vi "setup-cs-scan-fpga.vi"(4 "state-machine-params":T5={"xy_settled_samples_threshold"=15, "xy_error_threshold"=0.01, "zup_err_threshold"=0.10000228881835938, "prescan_samples"=5000, "TOL"=0.3, "collect_all"=TRUE, "numEntities"=0} {"TOL" format="%#_13g"}, 5 "Control-matrices":sgl[](array[numeric]), 6 "log-channels":u16(ring) items=["without-friction"=5, "with-friction"=6], 7 "ControlParamsLin-ss":T2={"umax"=3.0, "Ns_obs/cntrl"=0, "du_max"=0.0, "Nbar"=0.0, "Nhyst"=0, "Nsat"=0, "Ndrift+1"=0, "Ki-y"=0.01, "Ns_xff+1"=0, "Ns_yff+1"=0, "Ns_Dx+1"=0, "Ns_Dy+1"=0, "Ki-x"=0.01}, 8 "error in":errorcluster, 10 "z_axis_params":T3={"z_u_max"=5.0, "setpoint_scan"=-0.3000030517578125, "Ki_scan"=0.02, "uz_safe"=0.0, "Kiz_down"=0.02, "setpoint_up"=-0.899993896484375, "do_Dz"=FALSE, "PID_while_xy_move"=FALSE, "TF_params"={"TF_order"=0, "Num"=[0.0, 0.0, 0.0, 0.0, 0.0, 0.0, 0.0, 0.0, 0.0], "Den"=[0.0, 0.0, 0.0, 0.0, 0.0, 0.0, 0.0, 0.0, 0.0]}, "KI_slope"=0.0, "enable_KI_sched"=FALSE, "KI_min"=0.0, "KI_max"=0.0} {"Kiz_down" format="%#_13g"; "Ki_scan" min=0 max=0.4 step=0.0025; "z_u_max" format="%#_13g"}, 11 "FPGA Interface in":T1) -> (0 "error out":errorcluster, 3 "FPGA Interface out":T1)   [LabVIEW 2017]
uses:
  <vilib>/rvi/interface/nirviMethod/nirviMethod.xnode
  <vilib>/FPGAPlugInAG/Dynamic/niLvFpga_ConfigureFifo_Dynamic.vi
  <vilib>/rvi/errors/niLvFpgaMergeErrorWithErrorCode.vi
  <vilib>/rvi/interface/nirviReadWriteControl/nirviReadWriteControl.xnode
  fpga_interface_lib/fpga_interface_types/cs-scan-inputs-TYPE.ctl
  fpga_interface_lib/fpga_interface.lvlib
  NiFpgaLv.dll
  <vilib>/Utility/error.llb/Error Cluster From Error Code.vi
  <vilib>/rvi/interface/Simulation/niFpgaSimulationCallBeginRW.vi
  <vilib>/rvi/errors/niLvFpgaAdjustHostInterfaceError.vi
  <vilib>/FPGAPlugInAG/Dynamic/niLvFpga_WriteFifo_Dynamic.vi
  fpga_VIs/controls/supervisor-params.ctl
  controls/TF-params.ctl
  controls/z-axis-params_v4_prescan.ctl
  fpga_VIs/fpga_subVIs_ssxy/fixed-point-ss/typeDefs/FXPControlParams-ss-xy.ctl
panel:
  out "Empty Elements Remaining":u32
  out "Actual Depth 3":u32
  out "Actual Depth 2":u32
  out "Actual Depth":u32
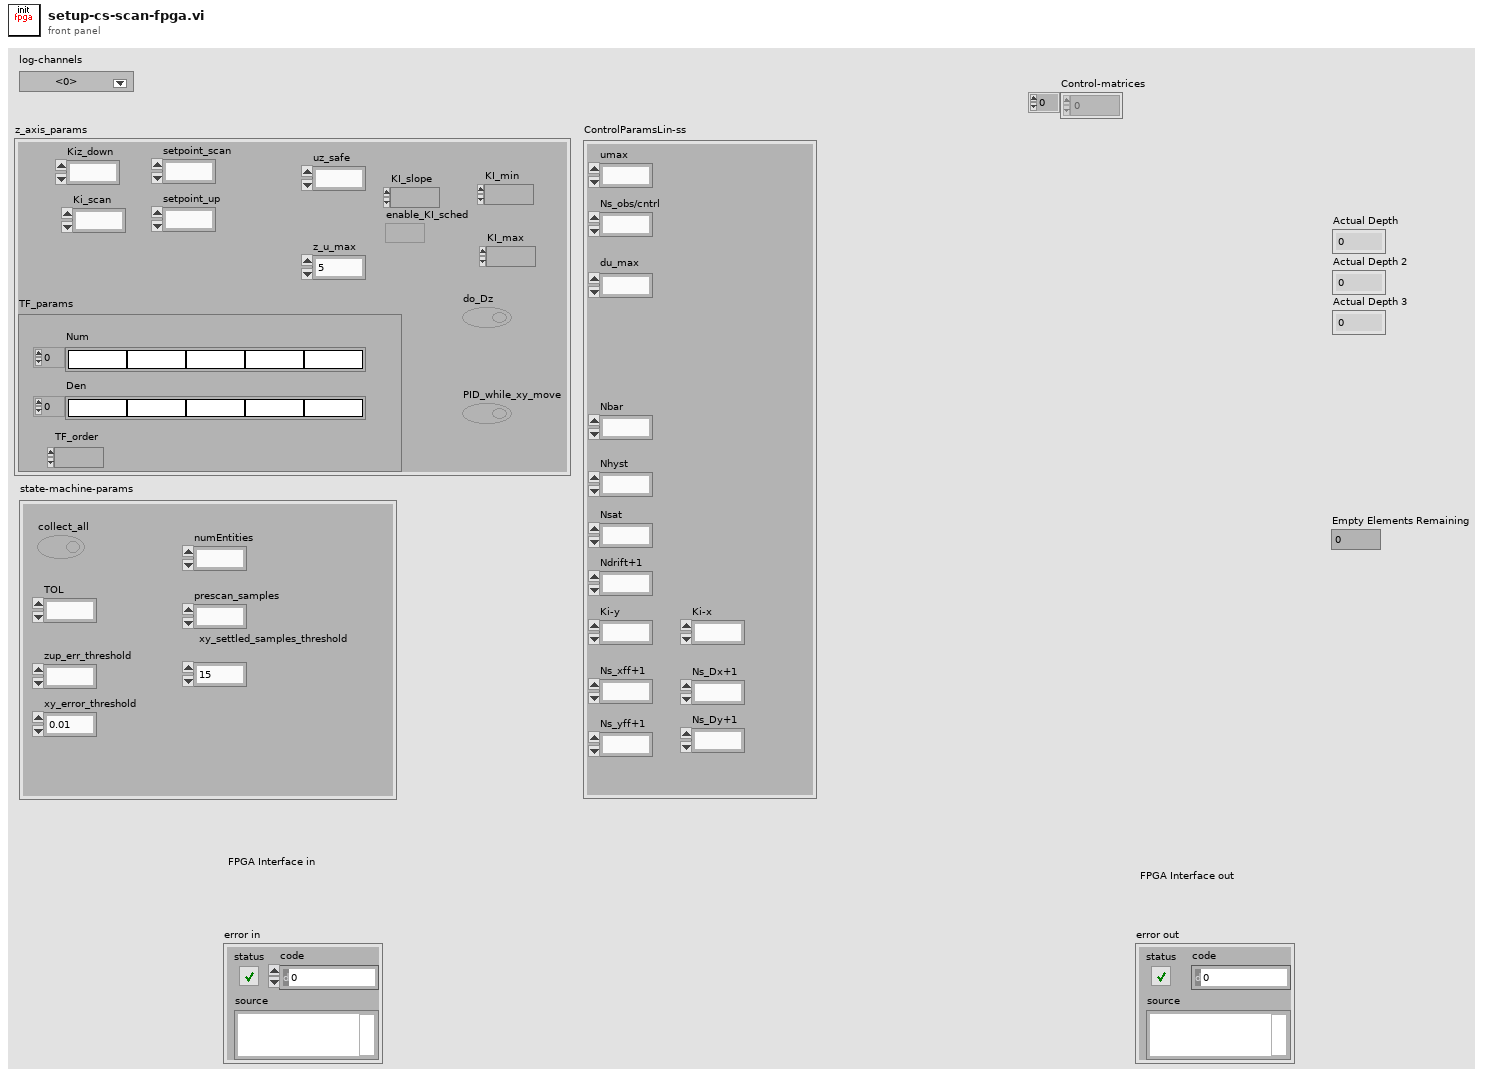
[diagram p1: front panel]
types:
  T1 = typedef "fpga_interface.lvlib/cs-scan-inputs-TYPE.ctl" = refnum<k20>
  T2 = typedef "FXPControlParams-ss-xy.ctl" = cluster{"umax":fxp<+/-,18,5>, "Ns_obs/cntrl":u8, "du_max":fxp<+/-,18,5>, "Nbar":fxp<+/-,32,5>, "Nhyst":u8, "Nsat":u8, "Ndrift+1":u8, "Ki-y":sgl, "Ns_xff+1":u8, "Ns_yff+1":u8, "Ns_Dx+1":u8, "Ns_Dy+1":u8, "Ki-x":sgl}
  T3 = typedef "z-axis-params_v4_prescan.ctl" = cluster{"z_u_max":sgl, "setpoint_scan":fxp<+/-,32,16>, "Ki_scan":sgl, "uz_safe":fxp<+/-,16,5>, "Kiz_down":sgl, "setpoint_up":fxp<+/-,32,16>, "do_Dz":bool, "PID_while_xy_move":bool, "TF_params":T4, "KI_slope":fxp<+/-,32,16>, "enable_KI_sched":bool, "KI_min":fxp<+/-,32,16>, "KI_max":fxp<+/-,32,16>}
  T4 = typedef "TF-params.ctl" = cluster{"TF_order":i16, "Num":sgl[], "Den":sgl[]}
  T5 = typedef "supervisor-params.ctl" = cluster{"xy_settled_samples_threshold":i16, "xy_error_threshold":sgl, "zup_err_threshold":fxp<+,24,5>, "prescan_samples":i16, "TOL":sgl, "collect_all":bool, "numEntities":i16}
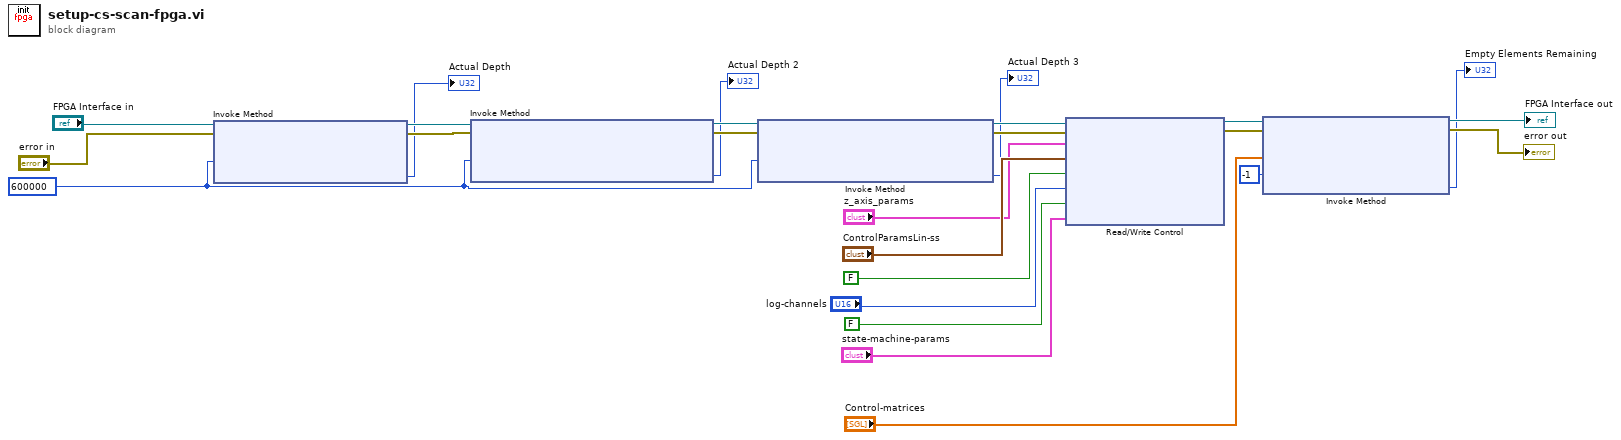
[diagram p0: block diagram]
diagram:
  w15 = 600000
  n1 = xnode "Invoke Method"("FPGA VI Reference In"="FPGA Interface in", "error in"="error in", "Requested Depth"=w15) -> ("FPGA VI Reference Out"=w19:T1, "error out"=w18:errorcluster, "Actual Depth"=→"Actual Depth":u32)
  n2 = xnode "Invoke Method"("FPGA VI Reference In"=w19, "error in"=w18, "Requested Depth"=w15) -> ("FPGA VI Reference Out"=w25:T1, "error out"=w24:errorcluster, "Actual Depth"=→"Actual Depth 2":u32)
  n3 = xnode "Invoke Method"("FPGA VI Reference In"=w25, "error in"=w24, "Requested Depth"=w15) -> ("FPGA VI Reference Out"=w23:T1, "error out"=w22:errorcluster, "Actual Depth"=→"Actual Depth 3":u32)
  n4 = xnode "Read/Write Control"("FPGA VI Reference In"=w23, "error in"=w22, "z_axis_params"="z_axis_params", "ControlParams-ss-xy"="ControlParamsLin-ss", "trigger-0"=FALSE, "num-log-channels"="log-channels", "ABORT"=FALSE, "state-machine-params"="state-machine-params") -> ("FPGA VI Reference Out"=w21:T1, "error out"=w20:errorcluster)
  n5 = xnode "Invoke Method"("FPGA VI Reference In"=w21, "error in"=w20, "Data"="Control-matrices", "Timeout (ms)"=-1) -> ("FPGA VI Reference Out"=→"FPGA Interface out":T1, "error out"=→"error out":errorcluster, "Empty Elements Remaining"=→"Empty Elements Remaining":u32)
